vi "SMU Switch Handshaking - LV code improvements.vi"(8 "error in":errorcluster, 11 "file path (use dialog)":path=path "C:/Users/IES/Desktop/jsontestfile.json") -> (0 "error out":errorcluster, 1 "Results":T1[](array[typedef]), 3 "Elapsed Time":u32)   [LabVIEW 2019]
uses:
  labview-grpc-query-server/VIs/MeasurementServer_FourProbeRawData.ctl
  labview-grpc-query-server/VIs/MeasurementServer_ErrorOutData.ctl
  <instrlib>/niDCPower/nidcpower.llb/niDCPower Send Software Edge Trigger - Signal.ctl
  <instrlib>/niDCPower/nidcpower.llb/niDCPower Configure Software Edge Start Trigger.vi
  <instrlib>/niDCPower/nidcpower.llb/niDCPower Configure Software Edge Sequence Advance Trigger.vi
  labview-grpc-query-server/VIs/labview-grpc-measurement-server.lvlib
  SupportVIs.lvlib
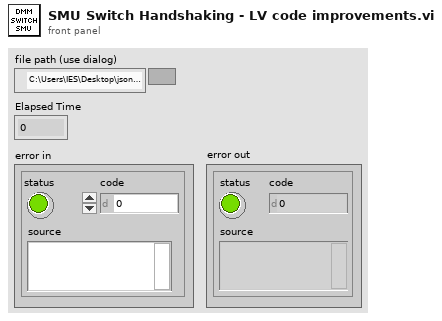
[diagram p1: front panel]
types:
  T1 = typedef "labview-grpc-measurement-server.lvlib/MeasurementServer_FourProbeRawData.ctl" = cluster{"Positive Voltage":sgl, "Positive Current":sgl, "Negative Voltage":sgl, "Negative Current":sgl, "Impedance":sgl, "ErrorOutData":T2}
  T2 = typedef "labview-grpc-measurement-server.lvlib/MeasurementServer_ErrorOutData.ctl" = cluster{"ErrorCode":i32, "ErrorMessage":string}
  T3 = typedef "niDCPower Send Software Edge Trigger - Signal.ctl" = i32
  T4 = typedef "JSONCluster.ctl" = cluster{"SMUResourceName":string, "SMUChannels":string, "SMUSourceMode_Sequence":i32, "SMUOutputFunction_DCCurrent":i32, "SMUSourceTransientResponse_Fast":i32, "SMUCurrent":dbl, "SMUCurrentLevelRange":dbl, "SMUMeasurementSense_Local":i32, "SMUMeasurementApertureTime":dbl, "SMUSourceAdvancedSourceDelay":dbl, "SMUVoltage":dbl, "SMUSourceAdvancedSequenceLoopCount":i32, "SMUMeasurementAdvancedDCNoiseRejection_Normal":i32, "SMUSequenceName":string, "SMUStep1_Source_DCCurrent_CurrentLevel":i32, "SMUStep2_Measurement_ApertureTime":i32, "SMUStep3_Source_Advanced_SourceDelay":i32, "SMUSequenceNumberOfSteps":i32, "SMUTriggerFromSwitch_StartDigitalEdge":string, "SMUTriggerFromSwitch_SequenceAdvanceDigitalEdge":string, "SMUTriggerToDMM_SourceCompleteEvent":i32, "SMUTriggerToDMM_SourceCompleteEvent_Value":string, "SMUTriggerToSwitch_SequenceIterationCompleteEvent":i32, "SMUTriggerToDMM_SequenceIterationCompleteEvent_Value":string, "Switch1ResourceName":string, "Switch1Topology":string, "Switch1ScanList":string, "Switch2ResourceName":string, "Switch2Topology":string, "Switch2ScanList":string, "DMMResourceName":string, "DMMFunction_DCVolts":i32, "DMMResolution":dbl, "DMMRange":dbl, "DMMTriggerSource_TTL2":i32, "DMMTriggerSlope_RisingEdge":i32, "DMMSampleTrigger_TTL2":i32, "DMMSampleCount":i32, "DMMSampleTriggerSlope_RisingEdge":i32, "DMMApertureTimeUnits_Seconds":i32, "DMMApertureTime":dbl, "DMMNumberOfAverages":i32, "DMMAutoZero_Off":i32, "DMMADCCalibration_Off":i32, "DMMSettleTime":dbl, "DMMControlAction_Commit":i32, "ApplicationNumberOfWeldChannels":i32}
  T5 = typedef "niDMM Acquisition State.ctl" = enum16{"Running", "Finished with Backlog", "Finished with no Backlog", "Paused", "No acquisition in progress"}
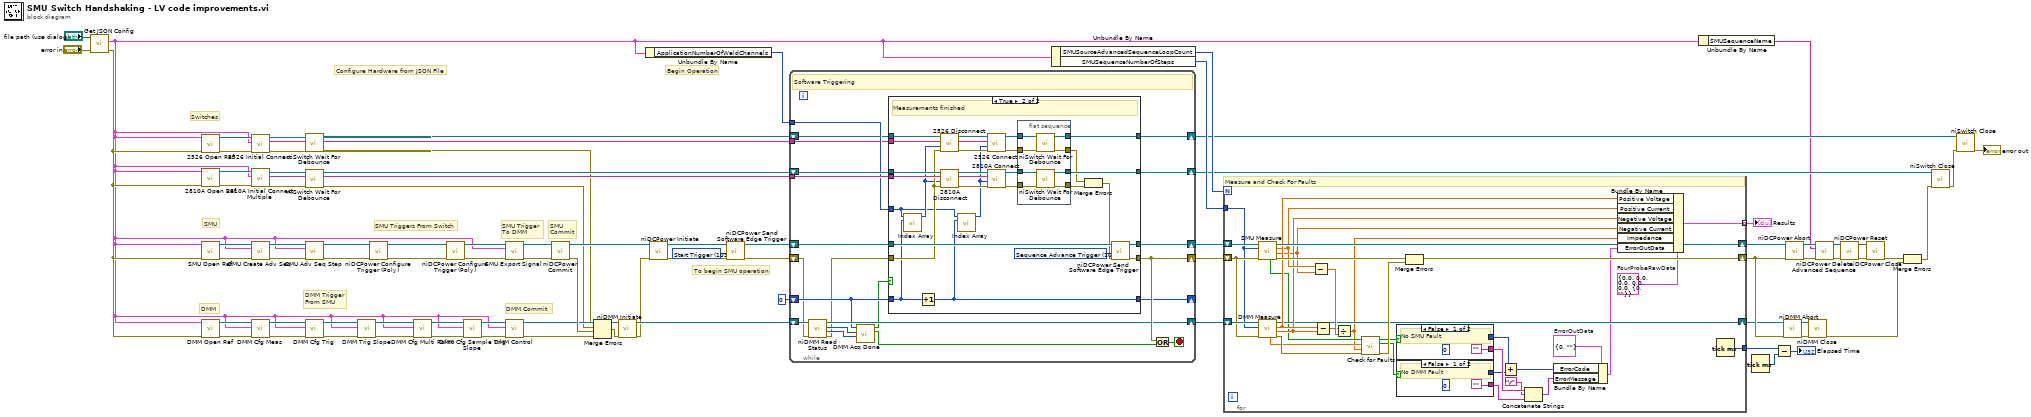
[diagram p0: block diagram]
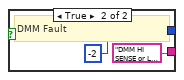
[diagram p3: hidden frame]
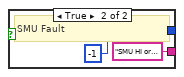
[diagram p4: hidden frame]
diagram:
  w31 = T3 1034 items=["Start Trigger"=1034, "Source Trigger"=1035, "Measure Trigger"=1036, "Sequence Advance Trigger"=1037, "Pulse Trigger"=1053] ("signal")
  # "SMU\nCommit"
  # "DMM Commit"
  # "Begin Operation"
  # "Configure Hardware from JSON File"
  # "DMM"
  # "SMU"
  # "Switches"
  # "To begin SMU operation"
  # "DMM Trigger\nFrom SMU"
  # "SMU Trigger \nTo DMM"
  # "SMU Triggers From Switch"
  n1 = call "Get JSON Config.vi"("error in (no error)"="error in", "JSON Configuration File (.json)"="file path (use dialog)") -> ("error out"=w2:errorcluster, "JSONCluster"=w1:T4)  [unwired: 6 in, 2 out]
  n2 = call "2526 Open Ref.vi"("error in"=w2, "JSONCluster"=w1) -> ("error out"=w15:errorcluster, "IVI Refnum out"=w16:refnum<k15>)  [unwired: 8 in]
  n3 = call "2810A Open Ref.vi"("error in"=w2, "JSONCluster"=w1) -> ("error out"=w22:errorcluster, "IVI Refnum out"=w23:refnum<k15>)  [unwired: 8 in]
  n4 = call "SMU Open Ref.vi"("error in (no error)"=w2, "JSONCluster"=w1) -> ("error out"=w83:errorcluster, "IVI Refnum out"=w84:refnum<k15>)  [unwired: 8 in]
  n5 = call "DMM Open Ref.vi"("error in"=w2, "JSONCluster"=w1) -> ("error out"=w56:errorcluster, "IVI Refnum out"=w55:refnum<k15>)  [unwired: 8 in]
  n6 = call "2526 Initial Connect.vi"("error in (no error)"=w15, "JSONCluster"=w1, "IVI Refnum in"=w16) -> ("error out"=w13:errorcluster, "2525 Scan List Channels"=w9:string[], "IVI Refnum out"=w14:refnum<k15>)  [unwired: 6 in]
  n7 = call "2810A Initial Connect Multiple.vi"("error in (no error)"=w22, "JSONCluster"=w1, "IVI Refnum in"=w23) -> ("error out"=w19:errorcluster, "Array"=w21:string[], "IVI Refnum out"=w20:refnum<k15>)  [unwired: 6 in]
  n8 = call "SMU Create Adv Seq.vi"("error in (no error)"=w83, "JSONCluster"=w1, "IVI Refnum in"=w84) -> ("error out"=w71:errorcluster, "IVI Refnum out"=w72:refnum<k15>)  [unwired: 7 in]
  n9 = call "DMM Cfg Meas.vi"("error in (no error)"=w56, "JSONCluster"=w1, "IVI Refnum in"=w55) -> ("error out"=w60:errorcluster, "IVI Refnum out"=w59:refnum<k15>)  [unwired: 7 in]
  n10 = call <instrlib>:"niSwitch Wait For Debounce.vi"("error in (no error)"=w13, "instrument handle"=w14) -> ("error out"=w11:errorcluster, "instrument handle out"=w10:refnum<k15>)  [unwired: 8 in]
  n11 = call <instrlib>:"niSwitch Wait For Debounce.vi"("error in (no error)"=w19, "instrument handle"=w20) -> ("error out"=w18:errorcluster, "instrument handle out"=w17:refnum<k15>)  [unwired: 8 in]
  n12 = call "SMU Adv Seq Step.vi"("error in (no error)"=w71, "JSONCluster"=w1, "IVI Refnum in"=w72) -> ("error out"=w69:errorcluster, "IVI Refnum out"=w70:refnum<k15>)  [unwired: 7 in]
  n13 = call "DMM Cfg Trig.vi"("error in (no error)"=w60, "JSONCluster"=w1, "IVI Refnum in"=w59) -> ("error out"=w62:errorcluster, "IVI Refnum out"=w61:refnum<k15>)  [unwired: 7 in]
  n14 = call "DMM Trig Slope.vi"("error in (no error)"=w62, "JSONCluster"=w1, "IVI Refnum in"=w61) -> ("error out"=w64:errorcluster, "IVI Refnum out"=w63:refnum<k15>)  [unwired: 7 in]
  n15 = call-poly <instrlib>:"niDCPower Configure Trigger (Poly).vi"("error in (no error)"=w69, "instrument handle"=w70) -> ("error out"=w80:errorcluster, "instrument handle out"=w81:refnum<k15>)  [unwired: 8 in]
  n16 = call "DMM Cfg Multi Point.vi"("error in (no error)"=w64, "JSONCluster"=w1, "IVI Refnum in"=w63) -> ("error out"=w66:errorcluster, "IVI Refnum out"=w65:refnum<k15>)  [unwired: 7 in]
  n17 = call-poly <instrlib>:"niDCPower Configure Trigger (Poly).vi"("error in (no error)"=w80, "instrument handle"=w81) -> ("error out"=w42:errorcluster, "instrument handle out"=w43:refnum<k15>)  [unwired: 8 in]
  n18 = call "DMM Cfg Sample Trig Slope.vi"("error in (no error)"=w66, "JSONCluster"=w1, "IVI Refnum in"=w65) -> ("error out"=w48:errorcluster, "IVI Refnum out"=w49:refnum<k15>)  [unwired: 7 in]
  n19 = call "SMU Export Signal.vi"("error in (no error)"=w42, "JSONCluster"=w1, "IVI Refnum in"=w43) -> ("error out"=w67:errorcluster, "IVI Refnum out"=w68:refnum<k15>)  [unwired: 7 in]
  n20 = call "DMM Control.vi"("error in (no error)"=w48, "JSONCluster"=w1, "IVI Refnum in"=w49) -> ("error out"=w53:errorcluster, "IVI Refnum out"=w50:refnum<k15>)  [unwired: 7 in]
  n21 = call <instrlib>:"niDCPower Commit.vi"("error in (no error)"=w67, "instrument handle"=w68) -> ("error out"=w54:errorcluster, "instrument handle out"=w51:refnum<k15>)  [unwired: 8 in]
  n22 = Merge Errors(w11, w18, w54, w53) -> (w52:errorcluster)
  n23 = call <instrlib>:"niDMM Initiate.vi"("error in (no error)"=w52, "instrument handle"=w50) -> ("error out"=w12:errorcluster, "instrument handle out"=w30:refnum<k15>)  [unwired: 8 in]
  n24 = Unbundle By Name(w1) -> ("ApplicationNumberOfWeldChannels"=w25:i32)
  n25 = call <instrlib>:"niDCPower Initiate.vi"("error in (no error)"=w12, "instrument handle"=w51) -> ("error out"=w24:errorcluster, "instrument handle out"=w34:refnum<k15>)  [unwired: 8 in]
  n26 = call <instrlib>:"niDCPower Send Software Edge Trigger.vi"("error in (no error)"=w24, "signal"=w31, "instrument handle"=w34) -> ("error out"=w32:errorcluster, "instrument handle out"=w33:refnum<k15>)  [unwired: 7 in]
  n27 = while {
    shift-right: [w105] -> w36
    shift-left: w33 -> [w100]
    shift-right: [w103] -> w35
    shift-left: w32 -> [w86]
    shift-right: [w101] -> w26
    shift-left: w17 -> [w102]
    shift-right: [w96] -> w29
    shift-left: w30 -> [w97]
    shift-right: [w94] -> _
    shift-left: 0 ("Backlog") -> [w95]
    tunnel: w21 -> [w91]
    tunnel: w25 -> [w90]
    shift-right: [w88] -> w8
    shift-left: w10 -> [w89]
    tunnel: w9 -> [w87]
    stop <- w104 stop-if-true
    # "Software Triggering"
    n28 = call <instrlib>:"niDMM Read Status.vi"("error in (no error)"=w86, "instrument handle"=w97) -> ("error out"=w85:errorcluster, "Acquisition State"=w99:T5, "Backlog"=w98:i32, "instrument handle out"=w96:refnum<k15>)  [unwired: 6 in]
    n29 = call "DMM Acq Done.vi"("Acquisition State"=w99, "Backlog"=w98, "Channel Index"=w95) -> ("Finished with Backlog?"=w93:bool, "Sequence Acquision Finished?"=w92:bool)  [unwired: 7 in]
    n30 = case shown="True" w92 {
      tunnel: w85 -> [w109 w119]
      tunnel: [w110 w137] -> w105
      tunnel: [w109 w136] -> w103
      tunnel: w100 -> [w110 w133]
      tunnel: w102 -> [w108 w132]
      tunnel: [w108 w135] -> w101
      tunnel: w95 -> [w107 w115]
      tunnel: [w107 w112] -> w94
      tunnel: w91 -> [_ w129]
      tunnel: w90 -> [_ w111]
      tunnel: w89 -> [w106 w124]
      tunnel: [w106 w121] -> w88
      tunnel: w87 -> [_ w120]
      frame False {
        # "Measurements not finished yet - repeat loop"
      }
      frame True {
        w134 = T3 1037 items=["Start Trigger"=1034, "Source Trigger"=1035, "Measure Trigger"=1036, "Sequence Advance Trigger"=1037, "Pulse Trigger"=1053] ("signal")
        # "Measurements finished"
        n31 = call "Index Array.vi"("Backlog"=w115, "ApplicationNumberOfWeldChannels"=w111) -> ("Index"=w114:i32)  [unwired: 9 in]
        n32 = Increment(x=w115) -> (x+1=w112:i32)
        n33 = call "2526 Disconnect.vi"("error in (no error)"=w119, "Index"=w114, "2525 Scan List Channels"=w120, "IVI Refnum in"=w124) -> ("error out"=w125:errorcluster, "IVI Refnum out"=w126:refnum<k15>)  [unwired: 6 in]
        n34 = call "2810A Disconnect.vi"("error in (no error)"=w119, "Numeric"=w114, "Array"=w129, "IVI Refnum in"=w132) -> ("error out"=w128:errorcluster, "IVI Refnum out"=w131:refnum<k15>)  [unwired: 6 in]
        n35 = call "Index Array.vi"("Backlog"=w112, "ApplicationNumberOfWeldChannels"=w111) -> ("Index"=w113:i32)  [unwired: 9 in]
        n36 = call "2526 Connect.vi"("error in (no error)"=w125, "Index"=w113, "2525 Scan List Channels"=w120, "IVI Refnum in"=w126) -> ("error out"=w122:errorcluster, "IVI Refnum out"=w123:refnum<k15>)  [unwired: 6 in]
        n37 = call "2810A Connect.vi"("error in (no error)"=w128, "Index"=w113, "Array"=w129, "IVI Refnum in"=w131) -> ("error out"=w127:errorcluster, "IVI Refnum out"=w130:refnum<k15>)  [unwired: 6 in]
        n38 = flat-sequence {
          tunnel: [w145] -> w135
          tunnel: [w144] -> w118
          tunnel: w130 -> [w143]
          tunnel: w127 -> [w142]
          tunnel: w123 -> [w141]
          tunnel: w122 -> [w140]
          tunnel: [w139] -> w121
          tunnel: [w138] -> w117
          frame #0 {
            n39 = call <instrlib>:"niSwitch Wait For Debounce.vi"("error in (no error)"=w140, "instrument handle"=w141) -> ("error out"=w138:errorcluster, "instrument handle out"=w139:refnum<k15>)  [unwired: 8 in]
            n40 = call <instrlib>:"niSwitch Wait For Debounce.vi"("error in (no error)"=w142, "instrument handle"=w143) -> ("error out"=w144:errorcluster, "instrument handle out"=w145:refnum<k15>)  [unwired: 8 in]
          }
        }
        n41 = Merge Errors(w117, w118) -> (w116:errorcluster)
        n42 = call <instrlib>:"niDCPower Send Software Edge Trigger.vi"("error in (no error)"=w116, "signal"=w134, "instrument handle"=w133) -> ("error out"=w136:errorcluster, "instrument handle out"=w137:refnum<k15>)  [unwired: 7 in]
      }
    }
    n43 = Or(x=w103, y=w93) -> (x .or. y?=w104:bool)
  }
  n44 = Unbundle By Name(w1) -> ("SMUSourceAdvancedSequenceLoopCount"=w38:i32, "SMUSequenceNumberOfSteps"=w37:i32)
  n45 = for {
    N: w38 -> [_]
    tunnel: w37 -> [w168]
    shift-right: [w175] -> w47
    shift-left: w35 -> [w169]
    shift-right: [w178] -> w82
    shift-left: w36 -> [w170]
    shift-right: [w163] -> w44
    shift-left: w29 -> [w177]
    tunnel: [w161] -> w5 mode=indexing
    tunnel: [w147] -> w3
    w148 = T2 {"ErrorCode"=0, "ErrorMessage"=""}  # ErrorOutData
    w146 = T1 {"Positive Voltage"=0.0, "Positive Current"=0.0, "Negative Voltage"=0.0, "Negative Current"=0.0, "Impedance"=0.0, "ErrorOutData"={"ErrorCode"=0, "ErrorMessage"=""}}  # FourProbeRawData
    # "Measure and Check For Faults"
    n46 = call "SMU Measure.vi"("error in (no error)"=w169, "SMUSequenceNumberOfSteps"=w168, "IVI Refnum in"=w170) -> ("error out"=w176:errorcluster, "Numeric"=w164:dbl, "Numeric 2"=w166:dbl, "IVI Refnum out"=w178:refnum<k15>, "in compliance"=w151:bool[])  [unwired: 4 in]
    n47 = call "DMM Measure.vi"("error in (no error)"=w169, "SMUSequenceNumberOfSteps"=w168, "IVI Refnum in"=w177) -> ("error out"=w174:errorcluster, "Numeric"=w165:dbl, "Numeric 2"=w167:dbl, "IVI Refnum out"=w163:refnum<k15>, "Measurements"=w150:dbl[])  [unwired: 4 in]
    n48 = Subtract(x=w166, y=w164) -> (x-y=w172:dbl)
    n49 = Subtract(x=w167, y=w165) -> (x-y=w171:dbl)
    n50 = Divide(x=w171, y=w172) -> (x/y=w149:dbl)
    n51 = call "Check for Faults.vi"("Error In"=w174, "Resistance In"=w149, "dmm voltage measurements"=w150, "in compliance"=w151) -> ("Error Out"=w173:errorcluster, "DMM Fault"=w155:bool, "SMU Fault"=w159:bool)  [unwired: 4 in, 1 out]
    n52 = case shown="False" w159 {
      tunnel: ["" "SMU HI or LO lead disconnected\n- SMU in compliance\n- SMU Fault = True"] -> w158
      tunnel: [0 -1] -> w156
      frame False {
        # "No SMU Fault"
      }
      frame True {
        # "SMU Fault"
      }
    }
    n53 = case shown="False" w155 {
      tunnel: ["" "DMM HI SENSE or LO SENSE lead disconnected\n- DMM measures NaN, or \n- DMM overrange warning, or\n- DMM voltage > 50uV "] -> w153
      tunnel: [0 -2] -> w152
      frame False {
        # "No DMM Fault"
      }
      frame True {
        # "DMM Fault"
      }
    }
    n54 = Merge Errors(w176, w173) -> (w175:errorcluster)
    n55 = Add(x=w156, y=w152) -> (x+y=w160:i32)
    n56 = Concatenate Strings(w158, "\r", w153) -> (w157:string)
    n57 = Bundle By Name(cluster=w148, "ErrorCode"=w160, "ErrorMessage"=w157) -> (w162:T2)
    n58 = Bundle By Name(cluster=w146, "Positive Voltage"=w167, "Positive Current"=w166, "Negative Voltage"=w165, "Negative Current"=w164, "Impedance"=w149, "ErrorOutData"=w162) -> (w161:T1)
    n59 = Tick Count (ms)() -> (millisecond timer value=w147:u32)
  }
  "Results" <- w5
  n60 = Unbundle By Name(w1) -> ("SMUSequenceName"=w4:string)
  n61 = Tick Count (ms)() -> (millisecond timer value=w79:u32)
  n62 = Subtract(x=w3, y=w79) -> (x-y=→"Elapsed Time":u32)
  n63 = call <instrlib>:"niDMM Abort.vi"("error in (no error)"=w47, "instrument handle"=w44) -> ("error out"=w58:errorcluster, "instrument handle out"=w57:refnum<k15>)  [unwired: 8 in]
  n64 = call <instrlib>:"niDCPower Abort.vi"("error in (no error)"=w47, "instrument handle"=w82) -> ("error out"=w77:errorcluster, "instrument handle out"=w78:refnum<k15>)  [unwired: 8 in]
  n65 = call <instrlib>:"niDMM Close.vi"("error in (no error)"=w58, "instrument handle"=w57) -> ("error out"=w46:errorcluster)  [unwired: 9 in]
  n66 = call <instrlib>:"niDCPower Delete Advanced Sequence.vi"("error in (no error)"=w77, "sequence name"=w4, "instrument handle"=w78) -> ("error out"=w76:errorcluster, "instrument handle out"=w75:refnum<k15>)  [unwired: 7 in]
  n67 = call <instrlib>:"niDCPower Reset.vi"("error in (no error)"=w76, "instrument handle"=w75) -> ("error out"=w73:errorcluster, "instrument handle out"=w74:refnum<k15>)  [unwired: 2 in, 6 out]
  n68 = call <instrlib>:"niDCPower Close.vi"("error in (no error)"=w73, "instrument handle"=w74) -> ("error out"=w45:errorcluster)  [unwired: 9 in]
  n69 = Merge Errors(w45, w46) -> (w27:errorcluster)
  n70 = call <instrlib>:"niSwitch Close.vi"("error in (no error)"=w27, "instrument handle"=w26) -> ("error out"=w7:errorcluster)  [unwired: 9 out]
  n71 = call <instrlib>:"niSwitch Close.vi"("error in (no error)"=w7, "instrument handle"=w8) -> ("error out"=→"error out":errorcluster)  [unwired: 9 out]
